vi "Read Aout Bias.vi"(8 "error in (no error)":errorcluster, 11 "VISA resource name":refnum<visa-resource-name>) -> (0 "error out":errorcluster, 2 "aout bias":cluster{"ABiasC":dbl, "ABiasL":dbl}, 3 "VISA resource name out":refnum<visa-resource-name>)   [LabVIEW 2020, in "Andeen-Hagerling 2700A.lvlib"]
doc: "The capacitance and loss analog outputs on the rear panel can\neach be fed from any one of three internal sources; the deviation\nsubsystem, the bias voltage source, or the zero voltage\nsource. This VI returns the output level produced by the\ncapacitance and/or loss bias voltage sources."
uses:
  Andeen-Hagerling 2700A.lvlib
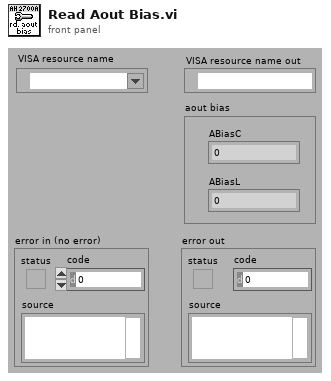
[diagram p1: front panel]
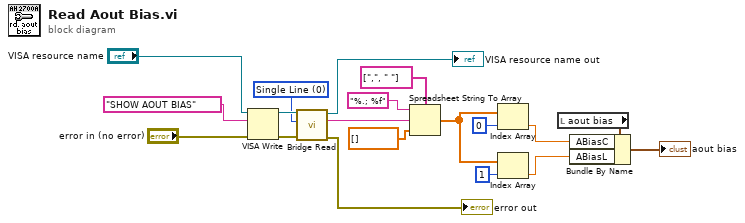
[diagram p0: block diagram]
diagram:
  w1 = u16 0 items=["Single Line", "Multi-Line"] ("Multiline")
  n1 = VISA Write(VISA resource name="VISA resource name", write buffer="SHOW AOUT BIAS" ("command"), error in (no error)="error in (no error)") -> (VISA resource name out=w6:refnum<visa-resource-name>, error out=w5:errorcluster)  [unwired: 1 out]
  n2 = call "Bridge Read.vi"("error in (no error)"=w5, "multiline"=w1, "VISA resource name"=w6) -> ("error out"=→"error out":errorcluster, "read buffer"=w2:string, "VISA resource name out"=→"VISA resource name out":refnum<visa-resource-name>)  [unwired: 6 in]
  n3 = Spreadsheet String To Array(delimiter (Tab)=string[] [",", " "], format string="%.; %f", spreadsheet string=w2, array type (2D Dbl)=dbl[] []) -> (array=w10:dbl[])
  n4 = Index Array(array=w10, index=0) -> (element=w8:dbl)
  n5 = Index Array(array=w10, index=1) -> (element=w9:dbl)
  n6 = local read "aout bias"() -> (w14:cluster{"ABiasC":dbl, "ABiasL":dbl})
  n7 = Bundle By Name(cluster=w14, "ABiasC"=w8, "ABiasL"=w9) -> (→"aout bias":cluster{"ABiasC":dbl, "ABiasL":dbl})
